vi "Dashboard Main.vi"() -> ()   [LabVIEW 2019]
uses:
  <vilib>/Utility/miscctls.llb/LVRowAndColumnTypeDef.ctl
  <vilib>/event_ctls.llb/eventvkey.ctl
  <vilib>/Rock Robotics/Network Tables/NT Read Numeric Array.vi
  <vilib>/Rock Robotics/WPI/Dashboard/WPI_DashboardLogging Global.vi
  <vilib>/Rock Robotics/Network Tables/NT Read Boolean.vi
panel:
  in  "Camera Settings Right":T1={"Frame Rate"=30, "Compression"=30, "Size"=1, "DB Camera Config"=FALSE} {"Frame Rate" scale=1.0..30.0; "Compression" scale=100.0..-1.0; "Size" items=["640x480", "320x240", "160x120"]}
  in  "Camera Name Right":string(combo)="No Camera Selection"
  out "Camera Perf":string
  in  "Camera Settings":T1={"Frame Rate"=30, "Compression"=30, "Size"=1, "DB Camera Config"=FALSE} {"Frame Rate" scale=1.0..30.0; "Compression" scale=100.0..-1.0; "Size" items=["640x480", "320x240", "160x120"]}
  in  "TCP":refnum<k5>
  in  "Rec Mode":enum32{"Stop", "Record", "Playback"}(radio)
  out "Robot IP":string
  out "Image Message":string="Timeout in Camera Communications"
  in  "Dashboard Tab":T2(tab)
  in  "FT to IN":bool
  out "Target Acquired":bool
  out "Vision Enabled":bool
  out "NT Connection":bool
  out "MotorChart R":cluster{"Numeric":dbl, "Numeric":dbl}(graph)
  out "MotorChart L":cluster{"Numeric":dbl, "Numeric":dbl}(graph)
  out "MotorSliders R":cluster{"MotorSlide1":dbl, "MotorSlide2":dbl} {"MotorSlide2" scale=-1.0..1.0 scale format="%#_2e"; "MotorSlide1" scale=-1.0..1.0 scale format="%#_2e"}
  out "MotorSliders L":cluster{"MotorSlide1":dbl, "MotorSlide2":dbl} {"MotorSlide2" scale=-1.0..1.0 scale format="%#_2e"; "MotorSlide1" scale=-1.0..1.0 scale format="%#_2e"}
  out "JS1 Z":dbl(slide) scale=-1.0..1.0 scale format="%#_2e"
  out "JS1 Graph":cluster{"X":dbl, "Y":dbl}[](graph)
  out "JS1 Buttons":T3
  out "JS2 Z":dbl(slide) scale=-1.0..1.0 scale format="%#_2e"
  out "JS2 Graph":cluster{"X":dbl, "Y":dbl}[](graph)
  out "JS2 Buttons":T3
  out "Mode":T4(ring)=enum."Auto Disabled"
  out "Right Camera Perf":cluster{"Bandwidth (Mbps)":dbl, "FPS":dbl}
  in  "Select Auto":string(combo)="Select Autonomous ..."
  out "Target Distance":dbl
  out "Camera Image Right":T5(plugin-control)
  out "Skew":dbl caption="DB/String 1"
  out "Area":dbl caption="DB/String 1"
  out "Offset X":dbl
  out "Offset Y":dbl
  out "Top RPM":dbl caption="DB/String 1"
  out "Bottom RPM":dbl caption="DB/String 1"
  in  "Test Slider":dbl(slide) scale=0.0..100.0 scale format="%#_3g"
  in  "On/Off":bool caption="Solenoid"
  in  "Test Name":u16(ring) items=["Select the test to run..."]
  in  "Test Tree":string(tree)
  in  "Motor":cluster{"Value":dbl, "Enable":bool} {"Value" scale=-1.0..1.0 scale format="%#_3g"}
  out "Progress":T6 {"Test Progress" scale=0.0..100.0}
  in  "Rev/Fwd":cluster{"Forward":bool, "Reverse":bool}
  in  "Test Ring":u16(ring) items=["Monochrome", "Color"]
  out "Cmd Status":string
  in  "Execute Command":bool
  in  "Command Params":string[][](table)
  in  "Command Selection":i32(listbox)
  in  "CheckList":i32(listbox)
  out "Tree":string(tree)
  out "Camera Image":T5(plugin-control)
  out "Background":bool
  in  "Camera Name":string(combo)="No Camera Selection"
  # "HW"
  # "HW"
  # "Drive Motors"
  # "Front"
  # "Operator 1"
  # "Operator 2"
  # "Right"
  # "Left"
  # "Back"
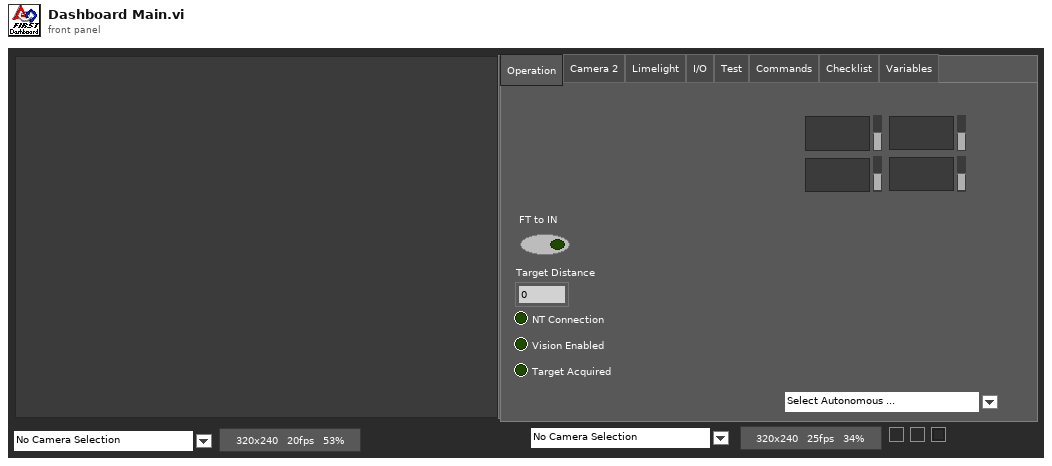
[diagram p1: front panel]
types:
  T1 = cluster{"Frame Rate":i32, "Compression":i32, "Size":u16, "DB Camera Config":bool}
  T2 = enum32{"Operation", "Camera 2", "Limelight", "I/O", "Test", "Commands", "Checklist", "Variables"}
  T3 = cluster{bool, bool, bool, bool, bool, bool, bool, bool, bool, bool, bool, bool}
  T4 = enum8{"Tele-Op Disabled", "Tele-Op Enabled", "Auto Disabled", "Auto Enabled", "Test Disabled", "Test Enabled", "Disconnected", "No Code", "E-Stop"}
  T5 = typedef "IMAQ Image.ctl" = refnum<image>
  T6 = cluster{"Test Progress":u8, "Test Progress Text":string}
  T7 = cluster{"Save Path":path, "Interval (s)":dbl, "Keep":i32}
  T8 = enum32{"Drive", "Camera", "Basic", "Custom", "Test", "Commands", "Checklist", "Variables"}
  T9 = typedef "Image Type" = u32
  T10 = cluster{"IDs":cluster{"RPC field ID":u16, "Unique ID":u16}, "String":string}
  T11 = cluster{"Camera Image":refnum<vi>, "Dashboard Tab":refnum<vi>, "Background":refnum<vi>, "Rec Mode":refnum<vi>, "Test Slider":refnum<vi>, "On/Off ":refnum<vi>, "Test Ring":refnum<vi>, "Rev/Fwd":refnum<vi>, "Test Name":refnum<vi>, "Motor":refnum<vi>, "Progress":refnum<vi>, "CheckList":refnum<vi>, "Tree":refnum<vi>, "Test Tree":refnum<vi>, "Command Params":refnum<vi>, "Command Selection":refnum<vi>, "Execute Command":refnum<vi>, "Cmd Status":refnum<vi>, "Camera Settings":refnum<vi>, "Camera Name":refnum<vi>, "Camera Perf":refnum<vi>, "Camera Settings Right":refnum<vi>, "Camera Name Right":refnum<vi>, "Camera Image Right":refnum<vi>}
  T12 = cluster{"Global Rectangle":i32[], "Contours":cluster{"Contour Type":u32, "ROI Type":u32, "Points":i32[]}[]}
  T13 = cluster{"Camera Name Right":string, string, "Saved DB Images Info":cluster{"Save Path":path, "Interval (s)":dbl, "Keep":i32}}
  T14 = cluster{"Error Strings":string, "Disable Counts":cluster{u16, u16}, "Rail Faults":cluster{u16, u16, u16}, "Robot IP":string, "DB Mode":u8, "Event Info":cluster{"Name":string, "Type":u8, "Number":u16, "Replay":u8}}
  T15 = cluster{"Storage":cluster{"Disk Free":u64, "RAM Block":u32, "RAM free":u32}, "CPU Utilization":cluster{"CPU % ISR":sgl, "CPU % Time Crit":sgl, "CPU % Timed Str":sgl, "CPU % High":sgl, "CPU % Above":sgl, "CPU % Normal":sgl, "CPU % Low":sgl}, "CAN":cluster{"% Bus Utilization":sgl, "Bus Off Cnt":u32, "TX_FIFO Full Cnt":u32, "Receive Error Cnt":u8, "Transmit Error Cnt":u8}, "HID":cluster{"HID Outputs":u32, "Rumble Low":u16, "Rumble High":u16}[]}
  T16 = cluster{"Status bits":cluster{"Test Mode":bool, "Autonomous":bool, "Enabled":bool, "Code Start":bool, "Brownout":bool, "Reserved 2":bool, "Reserved 3":bool, "E-Stop":bool}, "Code Trace":cluster{"Disabled":bool, "TeleOp":bool, "Auto":bool, "Test":bool}, "Controller Type":enum16{"unknown", "cRIO", "roboRio"}, "Code?":enum16{"unknown", "noCode", "code"}, "Battery V":dbl}
  T17 = cluster{"Control Bits":cluster{"TestMode":bool, "Autonomous":bool, "Enabled":bool, "FMS Present":bool, bool, bool, bool, "E-Stop":bool}, "Team Station ":u8, "Countdown":sgl, "Joystick Values":cluster{"Axes":dbl[], "Buttons":bool[], "POVs":i16[]}[]}
  T18 = cluster{"Axes":dbl[], "Buttons":bool[], "POVs":i16[]}[]
  T19 = cluster{"Axes":dbl[], "Buttons":bool[], "POVs":i16[]}
  T20 = cluster{"Buttons[0]":bool, "Buttons[1]":bool, "Buttons[2]":bool, "Buttons[3]":bool, "Buttons[4]":bool, "Buttons[5]":bool, "Buttons[6]":bool, "Buttons[7]":bool, "Buttons[8]":bool, "Buttons[9]":bool, "Buttons[10]":bool, "Buttons[11]":bool}
  T21 = cluster{"Camera Name":string, string, "Saved DB Images Info":cluster{"Save Path":path, "Interval (s)":dbl, "Keep":i32}}
  T22 = cluster{"Operation":enum16{"Update", "Clear"}, "Color Box":u32}[]
  T23 = typedef "eventvkey.ctl" = enum16{"ASCII", "Enter", "Return", "Shift", "Ctrl", "Alt", "Cmd", "Opt", "Caps", "NumLock", "Clear", "Break", "Up", "Down", "Left", "Right", "Insert", "Delete", "Home", "End", "PageUp", "PageDown", "Escape", "Help", "Pause", "ScrollLock", "F1", "F2", "F3", "F4", "F5", "F6", "F7", "F8", "F9", "F10", "F11", "F12", "F13", "F14", "F15", "F16", "F17", "F18", "F19", "F20", "F21", "F22", "F23", "F24", "Play", "VolumeUp", "VolumeDown", "Mute", "Two Byte Char"}
  T24 = cluster{"Image Size":bool, "Image Type":bool, "Pixel Value":bool, "ROI Information":bool, "Zoom Factor":bool}
  T25 = cluster{"Operation":enum16{"Update", "Clear"}, "Color Box":u32}
  T26 = typedef "LVRowAndColumnTypeDef.ctl" = cluster{"Row":i32, "Column":i32}
  T27 = cluster{"Shift":bool, "Ctrl":bool, "Alt":bool, "Cmd":bool, "Opt":bool}
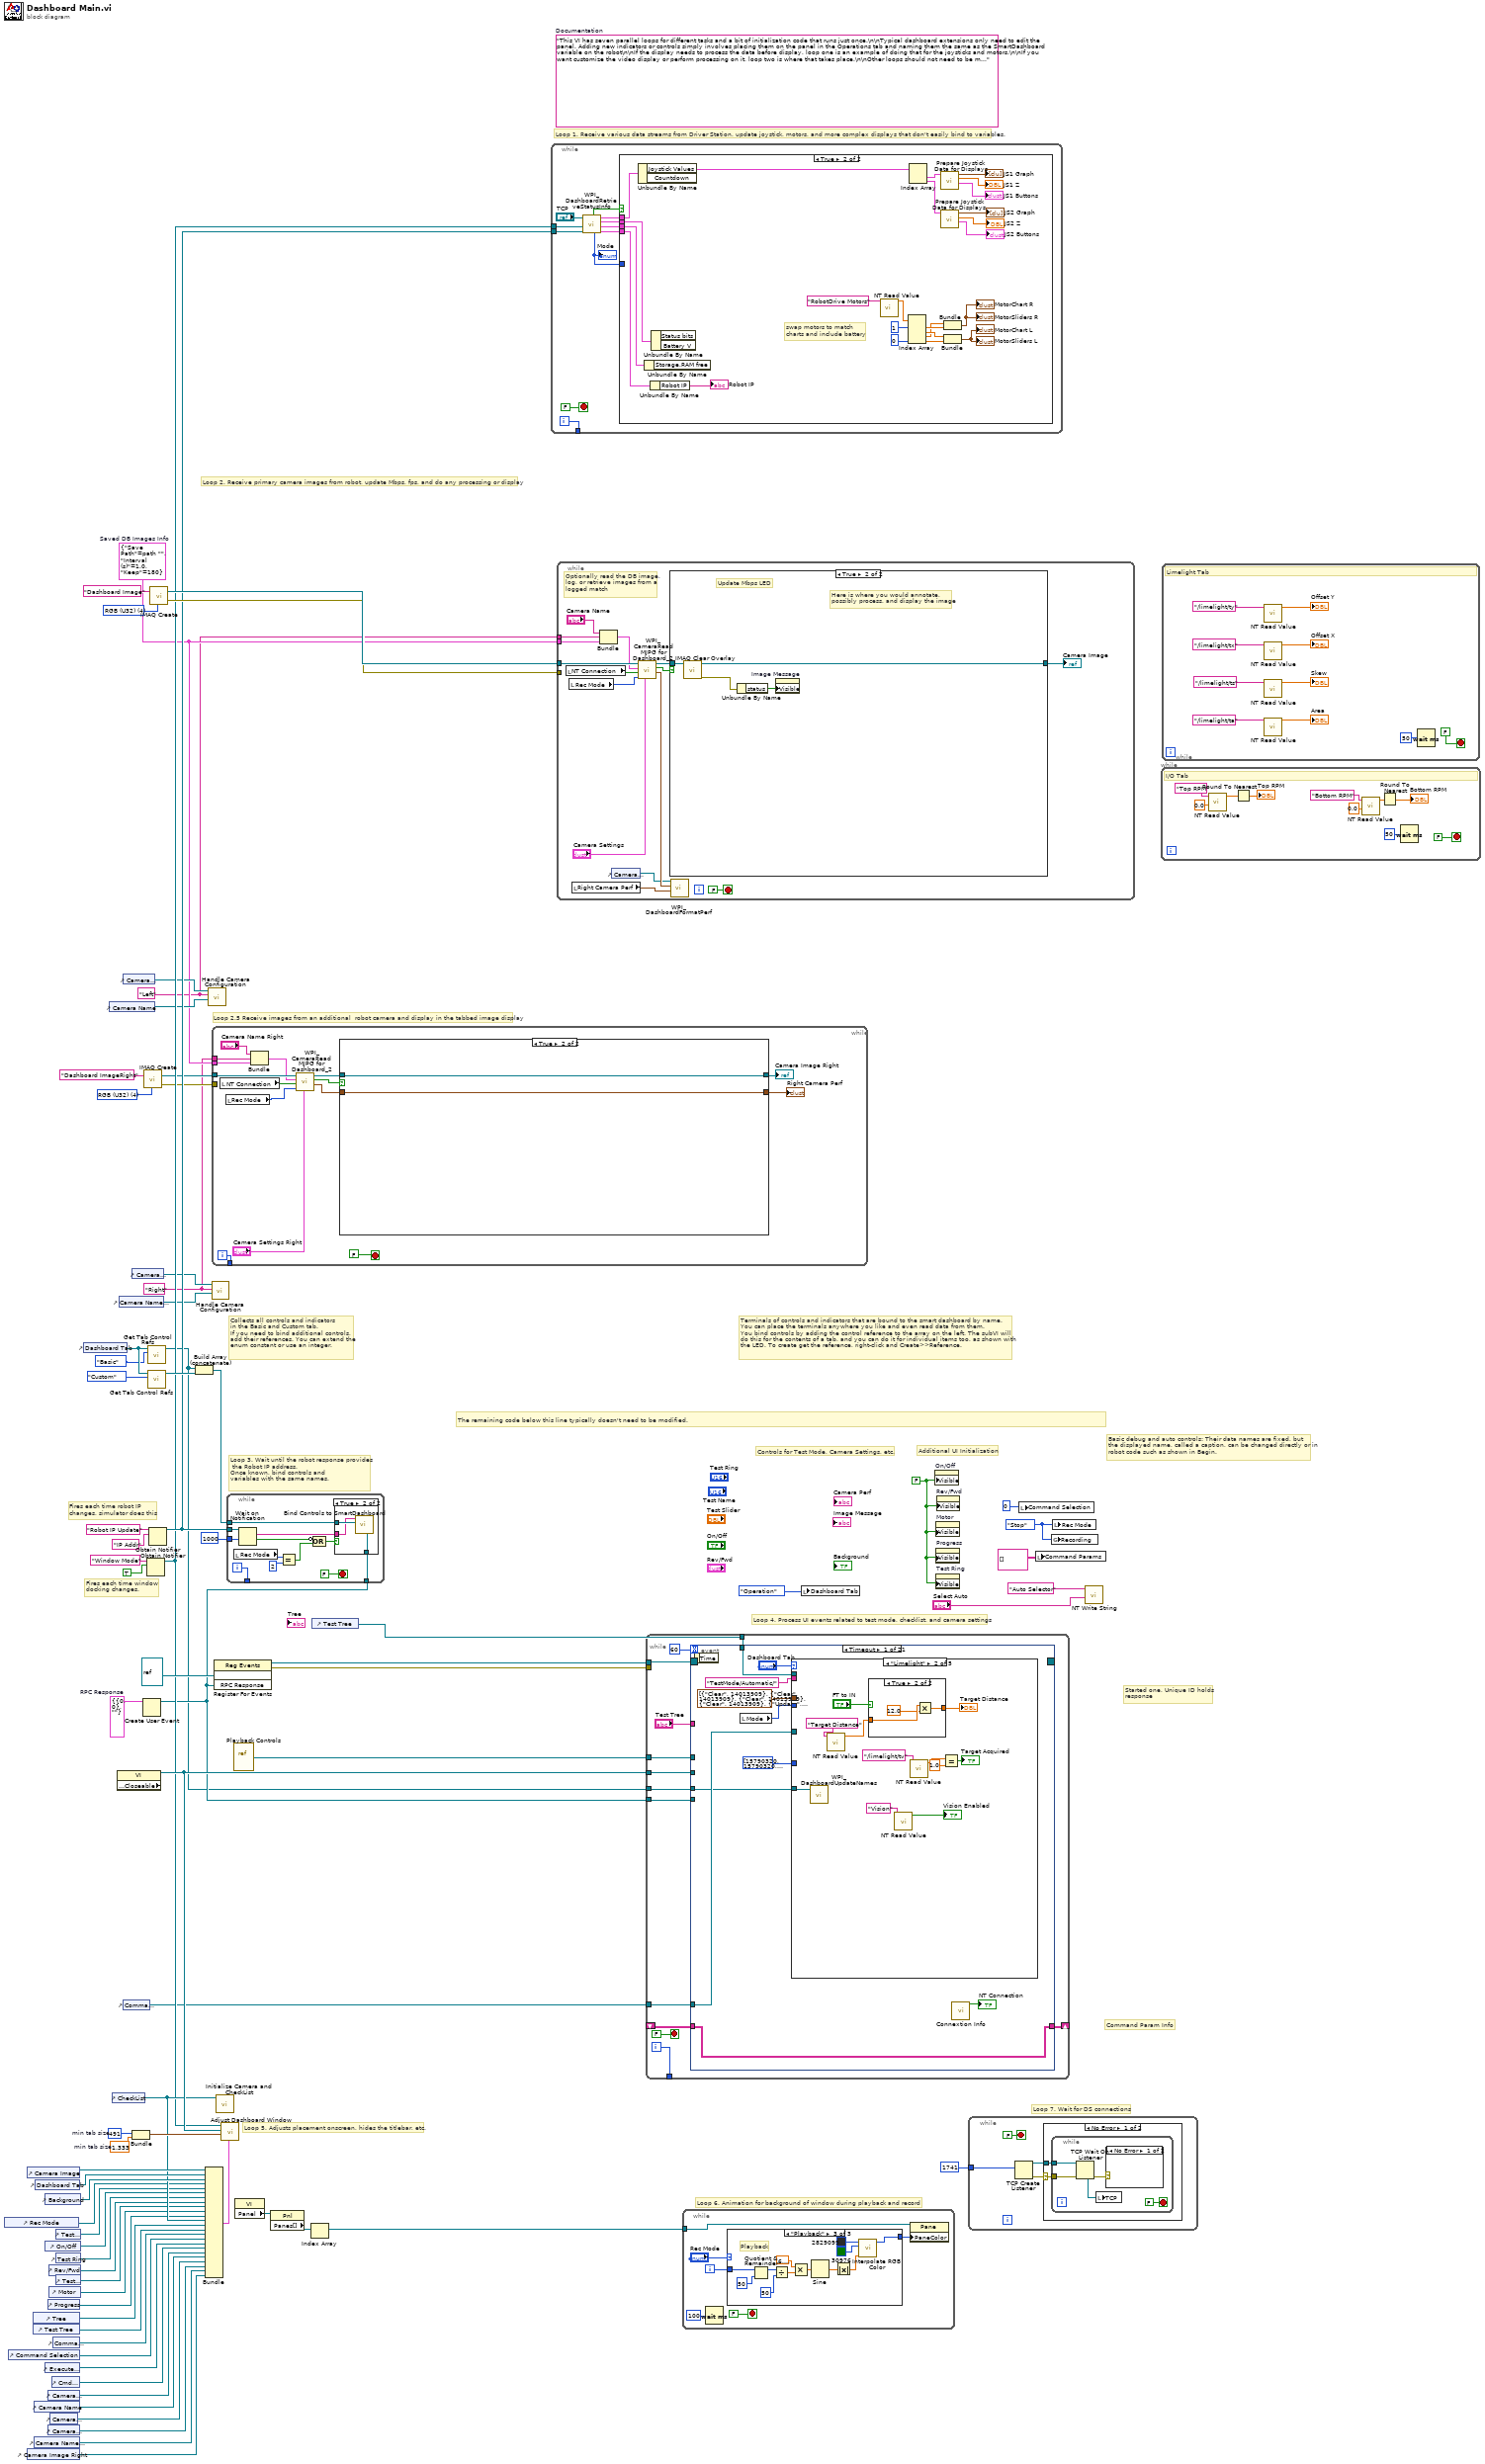
[diagram p0: block diagram]
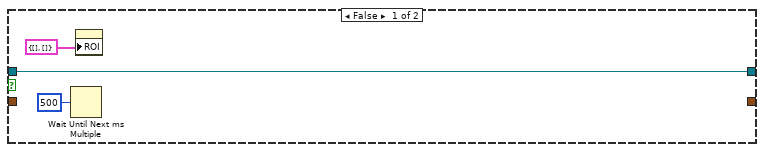
[diagram p2: hidden frame]
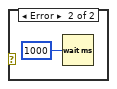
[diagram p3: hidden frame]
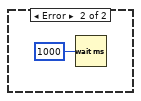
[diagram p4: hidden frame]
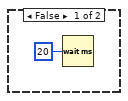
[diagram p5: hidden frame]
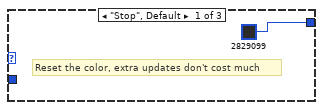
[diagram p6: hidden frame]
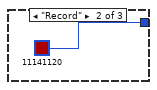
[diagram p7: hidden frame]
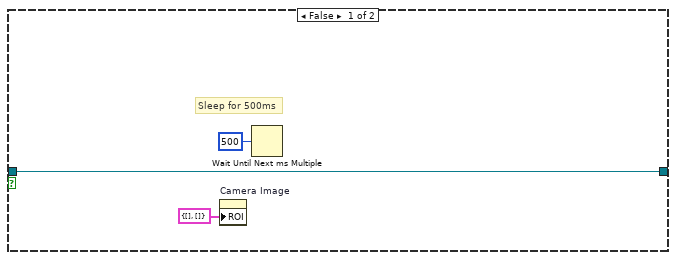
[diagram p9: hidden frame]
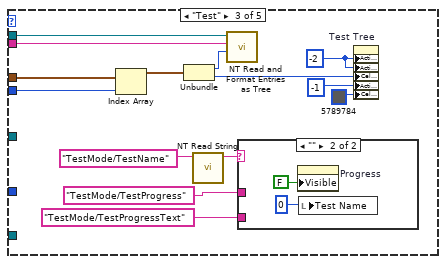
[diagram p12: hidden frame]
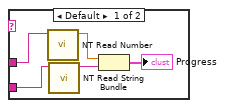
[diagram p13: hidden frame]
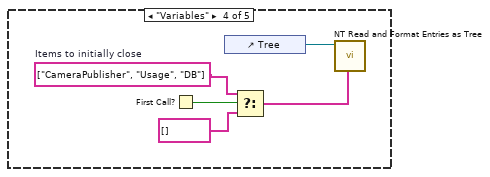
[diagram p14: hidden frame]
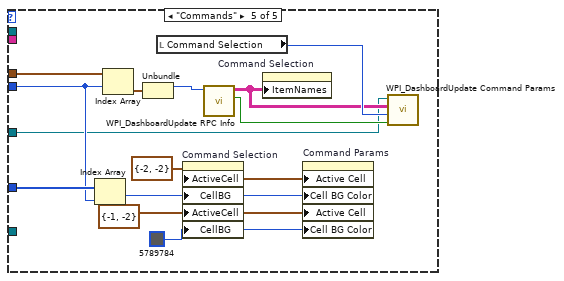
[diagram p15: hidden frame]
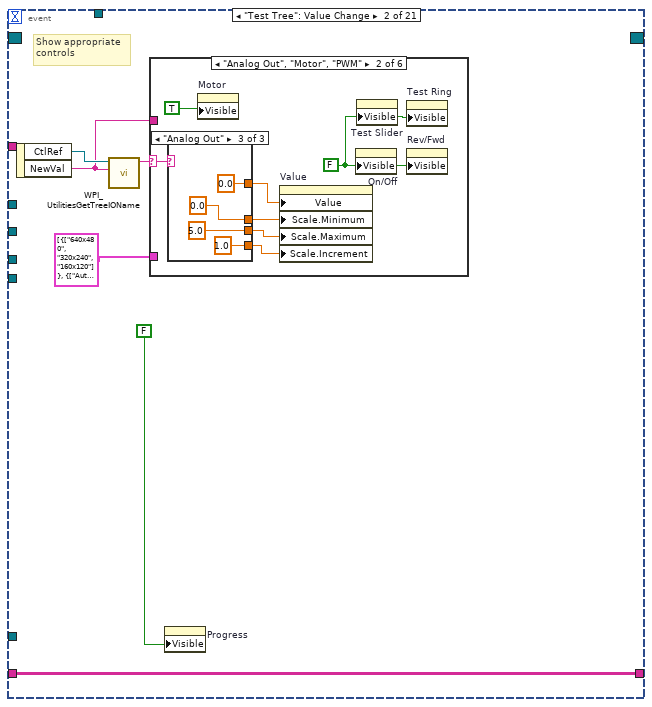
[diagram p16: hidden frame]
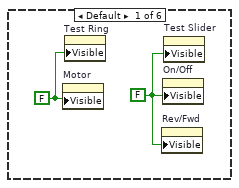
[diagram p17: hidden frame]
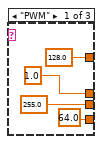
[diagram p18: hidden frame]
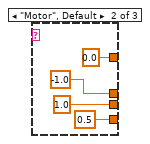
[diagram p19: hidden frame]
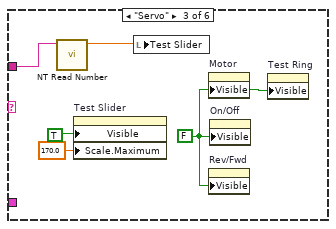
[diagram p20: hidden frame]
diagram:
  w4 = T7 {"Save Path"=path "", "Interval (s)"=1.0, "Keep"=180}  # Saved DB Images Info
  w3 = "Right"
  w2 = "Left"
  w14 = T9 4 items=["Grayscale (U8)", "Grayscale (I16)", "Grayscale (SGL)", "Complex (CSG)", "RGB (U32)", "HSL (U32)", "RGB (U64)"] ("Image Type")
  w30 = T10 {"IDs"={"RPC field ID"=0, "Unique ID"=0}, "String"=""}  # RPC Response
  w52 = 491  # min tab size
  w51 = 1.333  # min tab size
  w59 = enum32{"Stop", "Record", "Playback"}."Stop" ("Rec Mode")
  w36 = FALSE ("Visible")
  (unwired) "This VI has seven parallel loops for different tasks and a bit of initialization code that runs just once.\n\nTypical dashboard extensions only need to edit the panel. Adding new indicators or controls simply involves placing them on the panel in the Operations tab and naming them the same as the SmartDashboard variable on the robot\n\nIf the display needs to process the data before display, loop one is an example of doing that for the joysticks and motors.\n\nIf you want customize the video display or perform processing on it, loop two is where that takes place.\n\nOther loops should not need to be modified. They are pretty standard, and document the task they perform."  # Documentation
  w76 = T9 4 items=["Grayscale (U8)", "Grayscale (I16)", "Grayscale (SGL)", "Complex (CSG)", "RGB (U32)", "HSL (U32)", "RGB (U64)"] ("Image Type")
  # "Loop 2.5 Receive images from an additional  robot camera and display in the tabbed image display"
  # "Command Param Info"
  # "Started one, Unique ID holds\nresponse"
  # "Loop 7. Wait for DS connections"
  # "Basic debug and auto controls: Their data names are fixed, but\nthe displayed name, called a caption, can be changed directly or in\nrobot code such as shown in Begin."
  # "Controls for Test Mode, Camera Settings, etc."
  # "Additional UI Initialization"
  # "Loop 6. Animation for background of window during playback and record"
  # "Fires each time robot IP\nchanges, simulator does this"
  # "Fires each time window\ndocking changes."
  # "Collects all controls and indicators\nin the Basic and Custom tab.\nIf you need to bind additional controls,\nadd their references. You can extend the\nenum constant or use an integer."
  # "The remaining code below this line typically doesn't need to be modified."
  # "Loop 4. Process UI events related to test mode, checklist, and camera settings"
  # "Terminals of controls and indicators that are bound to the smart dashboard by name.\nYou can place the terminals anywhere you like and even read data from them.\nYou bind controls by adding the control reference to the array on the left. The subVI will\ndo this for the contents of a tab, and you can do it for individual items too, as shown with\nthe LED. To create get the reference, right-click and Create>>Reference."
  # "Loop 3. Wait until the robot response provides\n the Robot IP address.\nOnce known, bind controls and\nvariables with the same names."
  # "Loop 5. Adjusts placement onscreen, hides the titlebar, etc."
  # "Loop 1. Receive various data streams from Driver Station, update joystick, motors, and more complex displays that don't easily bind to variables."
  # "Loop 2. Receive primary camera images from robot, update Mbps, fps, and do any processing or display"
  n1 = control-ref of="Rec Mode"() -> (w42:refnum<vi>)
  n2 = control-ref of="Command Selection"() -> (w29:refnum<vi>)
  n3 = control-ref of="Camera Image Right"() -> (w7:refnum<vi>)
  n4 = control-ref of="Camera Image"() -> (w54:refnum<vi>)
  n5 = control-ref of="Tree"() -> (w46:refnum<vi>)
  n6 = control-ref of="Test Tree"() -> (w45:refnum<vi>)
  n7 = control-ref of="Camera Name"() -> (w20:refnum<vi>)
  n8 = control-ref of="Camera Name Right"() -> (w8:refnum<vi>)
  n9 = control-ref of="Dashboard Tab"() -> (w53:refnum<vi>)
  n10 = control-ref of="Execute Command"() -> (w31:refnum<vi>)
  n11 = control-ref of="Background"() -> (w49:refnum<vi>)
  n12 = control-ref of="On/Off"() -> (w40:refnum<vi>)
  n13 = control-ref of="Progress"() -> (w37:refnum<vi>)
  n14 = control-ref of="Camera Settings"() -> (w21:refnum<vi>)
  n15 = control-ref of="Camera Settings Right"() -> (w9:refnum<vi>)
  n16 = control-ref of="Rev/Fwd"() -> (w38:refnum<vi>)
  n17 = control-ref of="Motor"() -> (w43:refnum<vi>)
  n18 = control-ref of="Camera Perf"() -> (w19:refnum<vi>)
  n19 = control-ref of="Cmd Status"() -> (w25:refnum<vi>)
  n20 = control-ref of="Command Params"() -> (w32:refnum<vi>)
  n21 = control-ref of="Test Slider"() -> (w41:refnum<vi>)
  n22 = control-ref of="Test Ring"() -> (w39:refnum<vi>)
  n23 = control-ref of="Test Name"() -> (w44:refnum<vi>)
  n24 = control-ref of="Dashboard Tab"() -> (w57:refnum<vi>)
  n25 = control-ref of="Camera Name"() -> (w22:refnum<vi>)
  n26 = control-ref of="CheckList"() -> (w47:refnum<vi>)
  n27 = property class="VI" props=["Front Panel.Closeable"]() -> (reference out=w58:refnum<vi>)  [unwired: 2 in, 2 out]
  n28 = control-ref of="Camera Name Right"() -> (w10:refnum<vi>)
  n29 = control-ref of="Camera Settings"() -> (w23:refnum<vi>)
  n30 = control-ref of="Command Params"() -> (w24:refnum<vi>)
  n31 = control-ref of="Camera Settings Right"() -> (w11:refnum<vi>)
  n32 = Bundle("min tab size"=w52, "min tab size"=w51) -> (w50:cluster{"min tab size":i32, "min tab size":dbl})  [unwired: 1 in]
  n33 = Create User Event(user event datatype=w30) -> (user event=w26:refnum<user-event>)  [unwired: 1 in, 1 out]
  n34 = call "IMAQ Create"("Image Name"="Dashboard ImageRight", "Image Type"=w14) -> ("New Image"=w13:T5, "error out"=w12:errorcluster)  [unwired: 2 in, 1 out]
  n35 = Obtain Notifier(name (unnamed)="Window Mode", notification data type=TRUE) -> (notifier out=w34:refnum<notifier>)  [unwired: 2 in, 2 out]
  n36 = call <vilib>:"Get Tab Control Refs.vi"("Page Index"=T8."Basic" ("Dashboard Tab"), "TabControl in"=w57) -> ("ControlsOnPage"=w18:refnum<vi>[])  [unwired: 9 in]
  n37 = call <vilib>:"Get Tab Control Refs.vi"("Page Index"=T8."Custom" ("Dashboard Tab"), "TabControl in"=w57) -> ("ControlsOnPage"=w56:refnum<vi>[])  [unwired: 9 in]
  n38 = Obtain Notifier(name (unnamed)="Robot IP Update", notification data type="IP Addr" ("name (unnamed)")) -> (notifier out=w35:refnum<notifier>)  [unwired: 2 in, 2 out]
  n39 = call "IMAQ Create"("Image Name"="Dashboard Image", "Image Type"=w76) -> ("New Image"=w74:T5, "error out"=w73:errorcluster)  [unwired: 2 in, 1 out]
  n40 = Build Array (concatenate)(w18, w56) -> (w55:refnum<vi>[])
  n41 = Bundle("Camera Image"=w54, "Dashboard Tab"=w53, "Background"=w49, "Rec Mode"=w42, "Test Slider"=w41, "On/Off"=w40, "Test Ring"=w39, "Rev/Fwd"=w38, "Test Name"=w44, "Motor"=w43, "Progress"=w37, "CheckList"=w47, "Tree"=w46, "Test Tree"=w45, "Command Params"=w32, "Command Selection"=w29, "Execute Command"=w31, "Cmd Status"=w25, "Camera Settings"=w21, "Camera Name"=w20, "Camera Perf"=w19, "Camera Settings Right"=w9, "Camera Name Right"=w8, "Camera Image Right"=w7) -> (w48:T11)  [unwired: 1 in]
  n42 = call "Handle Camera Configuration.vi"("CameraNameRef"=w22, "Display Name"=w2, "ClusterRef"=w23) -> ()  [unwired: 9 in]
  n43 = call "Handle Camera Configuration.vi"("CameraNameRef"=w10, "Display Name"=w3, "ClusterRef"=w11) -> ()  [unwired: 9 in]
  n44 = while {
    tunnel: w13 -> [w91]
    tunnel: w12 -> [_]
    tunnel: [w86] -> _
    tunnel: w4 -> [w83]
    tunnel: w3 -> [w80]
    i -> [w86]
    stop <- FALSE stop-if-true
    n45 = local read "NT Connection"() -> (w84:bool)
    n46 = local read "Rec Mode"() -> (w90:enum32{"Stop", "Record", "Playback"})
    n47 = Bundle("Camera Name Right"="Camera Name Right", w80, "Saved DB Images Info"=w83) -> (w82:T13)  [unwired: 1 in]
    n48 = call <vilib>:"WPI_CameraRead MJPG for Dashboard_2.vi"("Camera Settings"="Camera Settings Right", "Rec Mode"=w90, "NT Connection"=w84, "Capture Info"=w82, "Image in"=w91) -> ("perf info"=w78:cluster{"Bandwidth (Mbps)":dbl, "fps":dbl}, "Active"=w85:bool, "Image\\ out"=w88:T5)  [unwired: 4 in]
    n49 = case shown="True" w85 {
      tunnel: w88 -> [w93 w95]
      tunnel: [w93 w95] -> w77
      tunnel: [_ w96] -> w79
      tunnel: w78 -> [_ w96]
      frame False {
        n50 = Wait Until Next ms Multiple(millisecond multiple=u32 500) -> ()  [unwired: 1 out]
        n51 = property on="Camera Image Right" class="ImageControl"("ROI"=T12 {"Global Rectangle"=[], "Contours"=[]}) -> ()  [unwired: 2 in, 2 out]
      }
      frame True {
      }
    }
    "Right Camera Perf" <- w79
    "Camera Image Right" <- w77
  }
  n52 = register-events(refnum<vi> refnum, w26) -> (reference out=w63:refnum<event-registration>, error out=w62:errorcluster)  [unwired: 2 in]
  n53 = call "Initialize Camera and CheckList.vi"("ListBox in"=w47) -> ()  [unwired: 11 in]
  n54 = call "Adjust Dashboard Window.vi"("Sizing Refnums"=w48, "Size Constraints"=w50, "VI"=w58, "WIn Mode"=w34) -> ()  [unwired: 8 in]
  n55 = while {
    tunnel: w55 -> [w108]
    tunnel: w35 -> [w106]
    tunnel: [w104] -> _
    tunnel: u32 1000 ("milliseconds to wait") -> [w103]
    tunnel: w26 -> [w97]
    i -> [w104]
    stop <- FALSE stop-if-true
    n56 = local read "Rec Mode"() -> (w99:enum32{"Stop", "Record", "Playback"})
    n57 = Wait on Notification(notifier=w106, timeout in ms (-1)=w103) -> (notification=w105:string, timed out?=w101:bool)  [unwired: 2 in, 2 out]
    n58 = Equal?(x=w99, y=u16 2 ("Rec Mode")) -> (x = y?=w100:bool)
    n59 = Compound Arithmetic op=OR(invert w101, w100) -> (w102:bool)
    n60 = case shown="True" w102 {
      tunnel: w108 -> [_ w111]
      tunnel: w105 -> [_ w110]
      tunnel: w97 -> [_ w109]
      frame False {
      }
      frame True {
        n61 = call <vilib>:"Bind Controls to SmartDashboard.vi"("RPC ref"=w109, "Bound Control Refs"=w111, "Server IP Address"=w110) -> ()  [unwired: 9 in]
      }
    }
  }
  n62 = vi-ref "Playback Controls.vi"() -> (w64:refnum<vi>)
  n63 = property class="VI"() -> ("Panel"=w66:refnum<vi>)  [unwired: 2 in, 2 out]
  n64 = property class="Pnl"(reference=w66) -> ("Panes[]"=w67:refnum<vi>[])  [unwired: 1 in, 2 out]
  n65 = Index Array(array=w67) -> (element=w65:refnum<vi>)  [unwired: 1 in]
  n66 = control-ref of="Test Tree"() -> (w68:refnum<vi>)
  n67 = while {
    tunnel: [w121] -> _
    tunnel: w35 -> [w115]
    tunnel: w34 -> [w112]
    i -> [w121]
    stop <- FALSE stop-if-true
    n68 = call <vilib>:"WPI_DashboardRetrieveStatusInfo.vi"("Binding Refnum"=w115, "Window Mode Notifier"=w112, "TCP Cnx"="TCP") -> ("Power and Errors"=w116:T14, "Robot Metrics"=w119:T15, "Status Info"=w120:T16, "Control Info"=w117:T17, "Robot Mode"=w114:T4, "Process?"=w118:bool)  [unwired: 3 in]
    "Mode" <- w114
    n69 = case shown="True" w118 {
      tunnel: w120 -> [_ w147]
      tunnel: w119 -> [_ w146]
      tunnel: w117 -> [_ w145]
      tunnel: w116 -> [_ w144]
      tunnel: w114 -> [_ _]
      frame False {
        n70 = Wait (ms)(milliseconds to wait=u32 20) -> ()  [unwired: 1 out]
      }
      frame True {
        # "swap motors to match\ncharts and include battery"
        n71 = Unbundle By Name(w145) -> ("Joystick Values"=w135:T18)  [unwired: 1 out]
        n72 = Unbundle By Name(w146) -> ()  [unwired: 1 out]
        n73 = Unbundle By Name(w144) -> ("Robot IP"=→"Robot IP":string)
        n74 = Unbundle By Name(w147) -> ()  [unwired: 2 out]
        n75 = call-poly <vilib>:"NT Read Value.vi"("Name"="RobotDrive Motors") -> ("Numeric Array"=w125:dbl[])  [unwired: 9 in, 1 out]
        n76 = Index Array(array=w125, index #1=1, index #4=0) -> (element #1=w139:dbl, element #2=w140:dbl, element #3=w138:dbl, element #4=w143:dbl)  [unwired: 2 in]
        n77 = Index Array(array=w135) -> (element #1=w134:T19, element #2=w130:T19)  [unwired: 2 in]
        n78 = call "Prepare Joystick Data for Displays.vi"("Joystick Values"=w130) -> ("Buttons"=→"JS2 Buttons":T20, "Z Axis"=→"JS2 Z":dbl, "Cartesian Data"=→"JS2 Graph":cluster{"X axis":dbl, "X axis":dbl}[])  [unwired: 8 in]
        n79 = call "Prepare Joystick Data for Displays.vi"("Joystick Values"=w134) -> ("Buttons"=→"JS1 Buttons":T20, "Z Axis"=→"JS1 Z":dbl, "Cartesian Data"=→"JS1 Graph":cluster{"X axis":dbl, "X axis":dbl}[])  [unwired: 8 in]
        n80 = Bundle("Numeric"=w138, "Numeric"=w139) -> (→"MotorChart R" →"MotorSliders R":cluster{"Numeric":dbl, "Numeric":dbl})  [unwired: 1 in]
        n81 = Bundle("Numeric"=w140, "Numeric"=w143) -> (→"MotorChart L" →"MotorSliders L":cluster{"Numeric":dbl, "Numeric":dbl})  [unwired: 1 in]
      }
    }
  }
  n82 = while {
    tunnel: w74 -> [w161]
    tunnel: w73 -> [_]
    tunnel: w4 -> [w155]
    tunnel: w2 -> [w152]
    stop <- FALSE stop-if-true
    # "Optionally read the DB image,\nlog, or retrieve images from a\nlogged match"
    n83 = local read "NT Connection"() -> (w156:bool)
    n84 = local read "Rec Mode"() -> (w158:enum32{"Stop", "Record", "Playback"})
    n85 = local read "Right Camera Perf"() -> (w150:cluster{"Bandwidth (Mbps)":dbl, "FPS":dbl})
    n86 = Bundle("Camera Name"="Camera Name", w152, "Saved DB Images Info"=w155) -> (w154:T21)  [unwired: 1 in]
    n87 = control-ref of="Camera Perf"() -> (w149:refnum<vi>)
    n88 = call <vilib>:"WPI_CameraRead MJPG for Dashboard_2.vi"("Camera Settings"="Camera Settings", "Rec Mode"=w158, "NT Connection"=w156, "Capture Info"=w154, "Image in"=w161) -> ("perf info"=w151:cluster{"Bandwidth (Mbps)":dbl, "fps":dbl}, "Active"=w159:bool, "Image\\ out"=w160:T5)  [unwired: 4 in]
    n89 = case shown="True" w159 {
      tunnel: w160 -> [w164 w167]
      tunnel: [w164 w166] -> w148
      frame False {
        # "Sleep for 500ms"
        n90 = property on="Camera Image" class="ImageControl"("ROI"=T12 {"Global Rectangle"=[], "Contours"=[]}) -> ()  [unwired: 2 in, 2 out]
        n91 = Wait Until Next ms Multiple(millisecond multiple=u32 500) -> ()  [unwired: 1 out]
      }
      frame True {
        # "Here is where you would annotate,\npossibly process, and display the image"
        # "Update Mbps LED"
        n92 = call "IMAQ Clear Overlay"("Image"=w167) -> ("error out"=w168:errorcluster, "Image Out"=w166:T5)  [unwired: 2 in, 7 out]
        n93 = Unbundle By Name(w168) -> ("status"=w169:bool)
        n94 = property on="Image Message" class="Str"("Visible"=w169) -> ()  [unwired: 2 in, 2 out]
      }
    }
    "Camera Image" <- w148
    n95 = call <vilib>:"WPI_DashboardFormatPerf.vi"("Right Camera Perf"=w150, "Performance"=w151, "String in"=w149) -> ()  [unwired: 9 in]
  }
  n96 = while {
    tunnel: [w179] -> _
    tunnel: w68 -> [w178]
    tunnel: w64 -> [w177]
    tunnel: w63 -> [w176]
    tunnel: w62 -> [_]
    tunnel: w58 -> [w175]
    tunnel: w26 -> [w174]
    tunnel: w24 -> [w173]
    shift-right: [w172] -> _
    shift-left: _ -> [w171]
    tunnel: w18 -> [w170]
    i -> [w179]
    stop <- FALSE stop-if-true
    n97 = event shown="[0] Timeout" {
      selector: w176 -> [_ _ _ _ _ _ _ _ _ _ _ _ _ _ _ _ _ _ _ _ _]
      dyn-events: [_ _ _ _ _ _ _ _ _ _ _ _ _ _ _ _ w453 _ _ _ _] -> _
      timeout: u32 60 ("milliseconds to wait") -> [_ _ _ _ _ _ _ _ _ _ _ _ _ _ _ _ _ _ _ _ _]
      tunnel: w178 -> [w191 _ _ _ _ _ _ _ _ _ _ _ _ _ _ _ _ _ _ _ _]
      tunnel: "Test Tree" -> [_ _ _ _ _ _ _ _ _ _ _ w420 w428 w430 w434 w442 _ _ _ _ _]
      tunnel: w177 -> [_ _ _ _ _ _ _ _ _ _ _ _ _ _ _ _ w455 _ w473 _ _]
      tunnel: w175 -> [_ _ _ _ _ _ _ _ _ _ _ _ _ _ _ _ w451 _ _ _ _]
      tunnel: w174 -> [_ _ _ _ _ _ _ _ _ _ _ _ _ _ _ _ w449 _ _ _ _]
      tunnel: w173 -> [w186 _ _ _ _ _ w371 _ _ _ _ _ _ _ _ _ _ _ _ _ _]
      tunnel: [w185 w248 w350 w355 w364 w368 w369 w378 w388 w395 w407 w419 w426 w429 w433 w441 w448 w468 w470 w474 w487] -> w172
      tunnel: w171 -> [w185 w248 w350 w355 w364 w368 w369 _ _ w395 w407 w419 w426 w429 w433 w441 w448 w468 w470 w474 w487]
      tunnel: w170 -> [w183 _ _ _ _ _ _ _ _ _ _ _ _ _ _ _ _ _ _ _ _]
      event Timeout {
        n98 = event-data() -> ()  [unwired: 1 in, 1 out]
        n99 = local read "Mode"() -> (w188:T4)
        n100 = case shown="\"Limelight\"" "Dashboard Tab" {
          tunnel: w191 -> [_ _ w221 _ _]
          tunnel: "TestMode/Automatic/" ("Name Pattern") -> [_ _ w220 _ _]
          tunnel: T22 [{"Operation"=enum."Clear", "Color Box"=14013909}, {"Operation"=enum."Clear", "Color Box"=14013909}, {"Operation"=enum."Clear", "Color Box"=14013909}, {"Operation"=enum."Clear", "Color Box"=14013909}, {"Operation"=enum."Update", "Color Box"=14013909}, {"Operation"=enum."Update", "Color Box"=16777215}, {"Operation"=enum."Clear", "Color Box"=14013909}, {"Operation"=enum."Clear", "Color Box"=14013909}, {"Operation"=enum."Clear", "Color Box"=14013909}] -> [_ _ w213 _ w241]
          tunnel: w188 -> [_ _ w212 _ w240]
          tunnel: u32[] [15790320, 15790320, 15790320, 15790320, 16777215, 16777215, 15790320, 15790320, 15790320] -> [_ _ _ _ w246]
          tunnel: w186 -> [_ _ _ _ w234]
          tunnel: w183 -> [_ w203 _ _ _]
          frame "I/O", Default {
          }
          frame "Limelight" {
            n101 = call <vilib>:"WPI_DashboardUpdateNames.vi"("Controls on Tab"=w203) -> ()  [unwired: 11 in]
            n102 = call-poly <vilib>:"NT Read Value.vi"("Name"="Target Distance") -> ("Numeric"=w201:dbl)  [unwired: 9 in, 1 out]
            n103 = case shown="True" "FT to IN" {
              tunnel: w201 -> [w204 w206]
              tunnel: [w204 w207] -> w202
              frame False {
              }
              frame True {
                n104 = Multiply(x=w206, y=12.0) -> (x*y=w207:dbl)
              }
            }
            "Target Distance" <- w202
            n105 = call-poly <vilib>:"NT Read Value.vi"("Name"="Vision") -> ("Boolean"=→"Vision Enabled":bool)  [unwired: 9 in, 1 out]
            n106 = call-poly <vilib>:"NT Read Value.vi"("Name"="/limelight/tv") -> ("Numeric"=w197:dbl)  [unwired: 9 in, 1 out]
            n107 = Equal?(x=w197, y=1.0) -> (x = y?=→"Target Acquired":bool)
          }
          frame "Test" {
            w219 = -2 ("Active Item:Row Number")
            n108 = Index Array(array=w213, index=w212) -> (element=w214:T25)
            n109 = Unbundle(w214) -> ("Operation"=w215:enum16{"Update", "Clear"}, "Color Box"=w216:u32)
            n110 = call <vilib>:"NT Read String.vi"("Name"="TestMode/TestName") -> ("String"=w210:string)  [unwired: 9 in, 1 out]
            n111 = call <vilib>:"NT Read and Format Entries as Tree.vi"("Operation"=w215, "Name Pattern"=w220, "Tree Refnum"=w221) -> ()  [unwired: 7 in, 2 out]
            n112 = case shown="\"\"" w210 {
              tunnel: "TestMode/TestProgress" ("Name") -> [w223 _]
              tunnel: "TestMode/TestProgressText" ("Name") -> [w222 _]
              frame Default {
                n113 = call <vilib>:"NT Read Number.vi"("Name"=w223) -> ("Numeric"=w224:dbl)  [unwired: 9 in, 1 out]
                n114 = call <vilib>:"NT Read String.vi"("Name"=w222) -> ("String"=w225:string)  [unwired: 9 in, 1 out]
                n115 = Bundle("Numeric"=w224, "String"=w225) -> (→"Progress":cluster{"Numeric":dbl, "String":string})  [unwired: 1 in]
              }
              frame "" {
                n116 = property on="Progress" class="Clust (strict)"("Visible"=FALSE) -> ()  [unwired: 2 in, 2 out]
                n117 = local write "Test Name"(u16 0) -> ()
              }
            }
            n118 = property on="Test Tree" class="Tree (strict)"("Active Item Row Number"=w219, "ActiveColNum"=w219, "CellBG"=w216, "Active Item Row Number"=-1 ("Active Item:Row Number"), "CellBG"=u32 5789784 ("Color Box")) -> ()  [unwired: 2 in, 2 out]
          }
          frame "Variables" {
            w231 = string[] ["CameraPublisher", "Usage", "DB"]  # Items to initially close
            n119 = First Call?() -> (First Call?: T/F=w232:bool)
            n120 = control-ref of="Tree"() -> (w233:refnum<vi>)
            n121 = Select(t=w231, s=w232, f=string[] []) -> (s? t:f=w229:string[])
            n122 = call <vilib>:"NT Read and Format Entries as Tree.vi"("Tags to  Close"=w229, "Tree Refnum"=w233) -> ()  [unwired: 8 in, 2 out]
          }
          frame "Commands" {
            w242 = u32 5789784 ("Color Box")
            w243 = T26 {"Row"=-1, "Column"=-2} ("Active Cell:Active Cell")
            w245 = T26 {"Row"=-2, "Column"=-2} ("Active Cell:Active Cell")
            n123 = Index Array(array=w246, index=w240) -> (element=w244:u32)
            n124 = Index Array(array=w241, index=w240) -> (element=w239:T25)
            n125 = Unbundle(w239) -> ("Operation"=w238:enum16{"Update", "Clear"})  [unwired: 1 out]
            n126 = local read "Command Selection"() -> (w237:i32)
            n127 = property on="Command Selection" class="MCListbox (strict)"("ActiveCell"=w245, "CellBG"=w244, "ActiveCell"=w243, "CellBG"=w242) -> ()  [unwired: 2 in, 2 out]
            n128 = call <vilib>:"WPI_DashboardUpdate RPC Info.vi"("Operation"=w238) -> ("update"=w236:bool, "commands"=w235:string[][])  [unwired: 9 in]
            n129 = property on="Command Selection" class="MCListbox (strict)"("ItemNames"=w235) -> ()  [unwired: 2 in, 2 out]
            n130 = property on="Command Params" class="Tbl (strict)"("Active Cell"=w245, "Cell BG Color"=w244, "Active Cell"=w243, "Cell BG Color"=w242) -> ()  [unwired: 2 in, 2 out]
            n131 = call <vilib>:"WPI_DashboardUpdate Command Params.vi"("Update"=w236, "NewVal"=w237, "Commands"=w235, "Param Tbl"=w234) -> ()  [unwired: 7 in, 1 out]
          }
        }
        n132 = call <vilib>:"Connextion Info.vi"() -> ("Connected"=→"NT Connection":bool)  [unwired: 10 in, 1 out]
      }
      event "Test Tree": Value Change {
        # "Show appropriate\ncontrols"
        n133 = event-data() -> ("CtlRef"=w251:refnum<vi>, "NewVal"=w249:string)  [unwired: 1 in]
        n134 = call <vilib>:"WPI_UtilitiesGetTreeIOName.vi"("NewVal"=w249, "TreeControl in"=w251) -> ("I/O Name"=w252:string)  [unwired: 9 in]
        n135 = case shown="\"Analog Out\", \"Motor\", \"PWM\"" w252 {
          selector: w252 -> [_ w259 _ w281 w290 _]
          tunnel: w249 -> [_ _ w278 w280 _ w297]
          tunnel: cluster{string[]}[] [{["640x480", "320x240", "160x120"]}, {["Auto", "Fixed indoor", "Fixed outdoor 1", "Fixed outdoor 2", "Fixed fluorescent 1", "Fixed fluorescent 2", "Hold current"]}, {["Auto", "Flicker-free 50 Hz", "Flicker-free 60 Hz", "Hold current"]}, {["None", "Prioritize frame rate", "Prioritize image quality"]}, {["Monochrome", "Color"]}] -> [_ _ _ _ _ w296]
          frame Default {
            w254 = FALSE ("Visible")
            w253 = FALSE ("Visible")
            n136 = property on="Motor" class="Clust (strict)"("Visible"=w253) -> ()  [unwired: 2 in, 2 out]
            n137 = property on="Test Ring" class="Ring (strict)"("Visible"=w253) -> ()  [unwired: 2 in, 2 out]
            n138 = property on="Rev/Fwd" class="Clust (strict)"("Visible"=w254) -> ()  [unwired: 2 in, 2 out]
            n139 = property on="On/Off" class="Bool (strict)"("Visible"=w254) -> ()  [unwired: 2 in, 2 out]
            n140 = property on="Test Slider" class="Slide (strict)"("Visible"=w254) -> ()  [unwired: 2 in, 2 out]
          }
          frame "Analog Out", "Motor", "PWM" {
            w260 = FALSE ("Visible")
            n141 = case shown="\"Analog Out\"" w259 {
              tunnel: [1.0 ("Value") -1.0 ("Value") 0.0 ("Value")] -> w258
              tunnel: [255.0 ("Value") 1.0 ("Value") 5.0 ("Value")] -> w257
              tunnel: [128.0 ("Value") 0.0 ("Value") 0.0 ("Value")] -> w256
              tunnel: [64.0 ("Value") 0.5 ("Value") 1.0 ("Value")] -> w255
              frame "PWM" {
              }
              frame "Motor", Default {
              }
              frame "Analog Out" {
              }
            }
            n142 = property on="Motor" class="Clust (strict)"("Visible"=TRUE) -> ()  [unwired: 2 in, 2 out]
            n143 = property on="Value" class="Slide (strict)"("Value"=w256, "Scale.Minimum"=w258, "Scale.Maximum"=w257, "Scale.Increment"=w255) -> ()  [unwired: 2 in, 2 out]
            n144 = property on="On/Off" class="Bool (strict)"("Visible"=w260) -> ()  [unwired: 2 in, 2 out]
            n145 = property on="Test Slider" class="Slide (strict)"("Visible"=w260) -> ()  [unwired: 2 in, 2 out]
            n146 = property on="Test Ring" class="Ring (strict)"("Visible"=w260) -> ()  [unwired: 2 in, 2 out]
            n147 = property on="Rev/Fwd" class="Clust (strict)"("Visible"=w260) -> ()  [unwired: 2 in, 2 out]
          }
          frame "Servo" {
            w276 = FALSE ("Visible")
            n148 = call <vilib>:"NT Read Number.vi"("Name"=w278) -> ("Numeric"=w277:dbl)  [unwired: 9 in, 1 out]
            n149 = property on="Test Slider" class="Slide (strict)"("Visible"=TRUE, "Scale.Maximum"=170.0 ("Scale.Range:Maximum")) -> ()  [unwired: 2 in, 2 out]
            n150 = local write "Test Slider"(w277) -> ()
            n151 = property on="Motor" class="Clust (strict)"("Visible"=w276) -> ()  [unwired: 2 in, 2 out]
            n152 = property on="Rev/Fwd" class="Clust (strict)"("Visible"=w276) -> ()  [unwired: 2 in, 2 out]
            n153 = property on="On/Off" class="Bool (strict)"("Visible"=w276) -> ()  [unwired: 2 in, 2 out]
            n154 = property on="Test Ring" class="Ring (strict)"("Visible"=w276) -> ()  [unwired: 2 in, 2 out]
          }
          frame "Relay", "Solenoid" {
            w279 = FALSE ("Visible")
            n155 = property on="Motor" class="Clust (strict)"("Visible"=w279) -> ()  [unwired: 2 in, 2 out]
            n156 = property on="Test Slider" class="Slide (strict)"("Visible"=w279) -> ()  [unwired: 2 in, 2 out]
            n157 = Search and Replace String(input string=w280, search string="/Value  **", replace string="/Direction") -> (result string=w286:string)  [unwired: 5 in, 3 out]
            n158 = property on="Test Ring" class="Ring (strict)"("Visible"=w279) -> ()  [unwired: 2 in, 2 out]
            n159 = call <vilib>:"NT Read String.vi"("Name"=w286) -> ("String"=w284:string)  [unwired: 9 in, 1 out]
            n160 = Equal?(x="Both directions", y=w284) -> (x = y?=w282:bool)
            n161 = Not(x=w282) -> (.not. x?=w283:bool)
            n162 = property on="Rev/Fwd" class="Clust (strict)"("Visible"=w282) -> ()  [unwired: 2 in, 2 out]
            n163 = property on="On/Off" class="Bool (strict)"("Visible"=w283, "Caption.Text"=w281) -> ()  [unwired: 2 in, 2 out]
          }
          frame "Compressor", "Digital Out" {
            w289 = FALSE ("Visible")
            # "Get direction and finish"
            n164 = property on="Motor" class="Clust (strict)"("Visible"=w289) -> ()  [unwired: 2 in, 2 out]
            n165 = property on="Test Slider" class="Slide (strict)"("Visible"=w289) -> ()  [unwired: 2 in, 2 out]
            n166 = property on="Test Ring" class="Ring (strict)"("Visible"=w289) -> ()  [unwired: 2 in, 2 out]
            n167 = property on="On/Off" class="Bool (strict)"("Visible"=TRUE, "Caption.Text"=w290) -> ()  [unwired: 2 in, 2 out]
            n168 = property on="Rev/Fwd" class="Clust (strict)"("Visible"=FALSE) -> ()  [unwired: 2 in, 2 out]
          }
          frame "Camera" {
            n169 = call <vilib>:"Get Last Path Segment.vi"("String in"=w297) -> ("String out"=w298:string)  [unwired: 10 in]
            n170 = property on="On/Off" class="Bool (strict)"("Visible"=FALSE) -> ()  [unwired: 2 in, 2 out]
            n171 = property on="Motor" class="Clust (strict)"("Visible"=FALSE) -> ()  [unwired: 2 in, 2 out]
            n172 = property on="Rev/Fwd" class="Clust (strict)"("Visible"=FALSE) -> ()  [unwired: 2 in, 2 out]
            n173 = case shown="\"White Balance  **\"" w298 {
              tunnel: w297 -> [w304 w313 w322 w331 w340 _ w346]
              tunnel: w296 -> [w302 w310 w319 w328 w337 _ _]
              frame "Size  **" {
                n174 = Index Array(array=w302) -> (element=w301:cluster{string[]})  [unwired: 1 in]
                n175 = call <vilib>:"NT Read String.vi"("Name"=w304) -> ("String"=w303:string)  [unwired: 9 in, 1 out]
                n176 = Unbundle(w301) -> (w299:string[])
                n177 = Match First String(2:w299, 3:w303) -> (0:w300:i32)  [unwired: 1 out]
                n178 = property on="Test Ring" class="Ring (strict)"("Value"=w300, "Strings []"=w299) -> ()  [unwired: 2 in, 2 out]
                n179 = property on="Test Ring" class="Ring (strict)"("Visible"=TRUE) -> ()  [unwired: 2 in, 2 out]
                n180 = property on="Test Slider" class="Slide (strict)"("Visible"=FALSE) -> ()  [unwired: 2 in, 2 out]
              }
              frame "White Balance  **" {
                n181 = Index Array(array=w310, index=1) -> (element=w311:cluster{string[]})
                n182 = call <vilib>:"NT Read String.vi"("Name"=w313) -> ("String"=w312:string)  [unwired: 9 in, 1 out]
                n183 = Unbundle(w311) -> (w308:string[])
                n184 = Match First String(2:w308, 3:w312) -> (0:w307:i32)  [unwired: 1 out]
                n185 = property on="Test Ring" class="Ring (strict)"("Value"=w307, "Strings []"=w308) -> ()  [unwired: 2 in, 2 out]
                n186 = property on="Test Ring" class="Ring (strict)"("Visible"=TRUE) -> ()  [unwired: 2 in, 2 out]
                n187 = property on="Test Slider" class="Slide (strict)"("Visible"=FALSE) -> ()  [unwired: 2 in, 2 out]
              }
              frame "Exposure  **" {
                n188 = Index Array(array=w319, index=2) -> (element=w320:cluster{string[]})
                n189 = call <vilib>:"NT Read String.vi"("Name"=w322) -> ("String"=w321:string)  [unwired: 9 in, 1 out]
                n190 = Unbundle(w320) -> (w316:string[])
                n191 = Match First String(2:w316, 3:w321) -> (0:w317:i32)  [unwired: 1 out]
                n192 = property on="Test Ring" class="Ring (strict)"("Value"=w317, "Strings []"=w316) -> ()  [unwired: 2 in, 2 out]
                n193 = property on="Test Ring" class="Ring (strict)"("Visible"=TRUE) -> ()  [unwired: 2 in, 2 out]
                n194 = property on="Test Slider" class="Slide (strict)"("Visible"=FALSE) -> ()  [unwired: 2 in, 2 out]
              }
              frame "Exposure Priority  **" {
                n195 = Index Array(array=w328, index=3) -> (element=w329:cluster{string[]})
                n196 = call <vilib>:"NT Read String.vi"("Name"=w331) -> ("String"=w330:string)  [unwired: 9 in, 1 out]
                n197 = Unbundle(w329) -> (w325:string[])
                n198 = Match First String(2:w325, 3:w330) -> (0:w326:i32)  [unwired: 1 out]
                n199 = property on="Test Ring" class="Ring (strict)"("Value"=w326, "Strings []"=w325) -> ()  [unwired: 2 in, 2 out]
                n200 = property on="Test Ring" class="Ring (strict)"("Visible"=TRUE) -> ()  [unwired: 2 in, 2 out]
                n201 = property on="Test Slider" class="Slide (strict)"("Visible"=FALSE) -> ()  [unwired: 2 in, 2 out]
              }
              frame "Color Enable  **" {
                n202 = Index Array(array=w337, index=4) -> (element=w338:cluster{string[]})
                n203 = call <vilib>:"NT Read String.vi"("Name"=w340) -> ("String"=w339:string)  [unwired: 9 in, 1 out]
                n204 = Unbundle(w338) -> (w334:string[])
                n205 = Match First String(2:w334, 3:w339) -> (0:w335:i32)  [unwired: 1 out]
                n206 = property on="Test Ring" class="Ring (strict)"("Value"=w335, "Strings []"=w334) -> ()  [unwired: 2 in, 2 out]
                n207 = property on="Test Ring" class="Ring (strict)"("Visible"=TRUE) -> ()  [unwired: 2 in, 2 out]
                n208 = property on="Test Slider" class="Slide (strict)"("Visible"=FALSE) -> ()  [unwired: 2 in, 2 out]
              }
              frame Default {
                n209 = property on="Test Ring" class="Ring (strict)"("Visible"=FALSE) -> ()  [unwired: 2 in, 2 out]
                n210 = property on="Test Slider" class="Slide (strict)"("Visible"=FALSE) -> ()  [unwired: 2 in, 2 out]
              }
              frame "Brightness  **", "Color Level  **", "Compression  **", "FPS  **", "Sharpness  **" {
                n211 = call <vilib>:"NT Read Number.vi"("Name"=w346) -> ("Numeric"=w345:dbl)  [unwired: 9 in, 1 out]
                n212 = local write "Test Slider"(w345) -> ()
                n213 = property on="Test Slider" class="Slide (strict)"("Visible"=TRUE, "Scale.Maximum"=100.0 ("Scale.Range:Maximum")) -> ()  [unwired: 2 in, 2 out]
                n214 = property on="Test Ring" class="Ring (strict)"("Visible"=FALSE) -> ()  [unwired: 2 in, 2 out]
              }
            }
          }
        }
        n215 = property on="Progress" class="Clust (strict)"("Visible"=FALSE) -> ()  [unwired: 2 in, 2 out]
      }
      event "Test Name": Mouse Enter {
        # "Populate the ring with the list of tests"
        n216 = event-data() -> ()  [unwired: 1 in, 1 out]
        n217 = call <vilib>:"NT Read String Array.vi"("Name"="TestMode/TestList") -> ("String Array"=w354:string[])  [unwired: 9 in, 1 out]
        n218 = Build Array (concatenate)("Select the test to run...", w354) -> (w353:string[])
        n219 = property on="Test Name" class="Ring (strict)"("Strings []"=w353) -> ()  [unwired: 2 in, 2 out]
      }
      event "Test Name": Value Change {
        w356 = FALSE ("Visible")
        # "Tell the robot the test name to run"
        n220 = event-data() -> ("NewVal"=w360:u16)  [unwired: 1 in]
        n221 = property on="Test Name" class="Ring (strict)"() -> ("Strings []"=w361:string[])  [unwired: 2 in, 2 out]
        n222 = local write "Progress"(T6 {"Test Progress"=0, "Test Progress Text"=""} ("Progress")) -> ()
        n223 = Index Array(array=w361, index=w360) -> (element=w359:string)
        n224 = call <vilib>:"NT Write String.vi"("String"=w359, "Name"="TestMode/TestName") -> ()  [unwired: 9 in, 1 out]
        n225 = property on="Progress" class="Clust (strict)"("Visible"=TRUE) -> ()  [unwired: 2 in, 2 out]
        n226 = property on="Motor" class="Clust (strict)"("Visible"=w356) -> ()  [unwired: 2 in, 2 out]
        n227 = property on="Test Slider" class="Slide (strict)"("Visible"=w356) -> ()  [unwired: 2 in, 2 out]
        n228 = property on="On/Off" class="Bool (strict)"("Visible"=w356) -> ()  [unwired: 2 in, 2 out]
        n229 = property on="Rev/Fwd" class="Clust (strict)"("Visible"=w356) -> ()  [unwired: 2 in, 2 out]
        n230 = property on="Test Ring" class="Ring (strict)"("Visible"=w356) -> ()  [unwired: 2 in, 2 out]
      }
      event "Select Auto": Mouse Enter {
        # "Populate the combo box with the list of autonomous options"
        n231 = event-data() -> ()  [unwired: 1 in, 1 out]
        n232 = call <vilib>:"NT Read String Array.vi"("Name"="Auto List") -> ("String Array"=w363:string[])  [unwired: 9 in, 1 out]
        n233 = property on="Select Auto" class="CmbBox"("Strings[]"=w363) -> ()  [unwired: 2 in, 2 out]
      }
      event "Select Auto": Value Change {
        # "User modified the Auto Selection. Write to NT variable so robot knows."
        n234 = event-data() -> ("NewVal"=w366:string)  [unwired: 1 in]
        n235 = call <vilib>:"NT Write String.vi"("String"=w366, "Name"="Auto Selector") -> ()  [unwired: 9 in, 1 out]
      }
      event "Command Selection": Value Change {
        # "Get the params and show in table"
        n236 = event-data() -> ("NewVal"=w372:i32)  [unwired: 1 in]
        n237 = property on="Command Selection" class="MCListbox (strict)"() -> ("ItemNames"=w370:string[][])  [unwired: 2 in, 2 out]
        n238 = call <vilib>:"WPI_DashboardUpdate Command Params.vi"("NewVal"=w372, "Commands"=w370, "Param Tbl"=w371) -> ()  [unwired: 8 in, 1 out]
      }
      event "Execute Command": Value Change {
        # "Started one, Unique ID holds\nresponse"
        n239 = event-data() -> ()  [unwired: 1 in, 1 out]
        n240 = property on="Command Selection" class="MCListbox (strict)"() -> ("ItemNames"=w383:string[][])  [unwired: 2 in, 2 out]
        n241 = Index Array(array=w383, index (row)="Command Selection", index (col)=0) -> (element=w381:string)
        n242 = call <vilib>:"Invoke Commands.vi"("Command Params"="Command Params", "Function Name"=w381) -> ("Params"=w377:u8, "Started"=w376:bool)  [unwired: 7 in, 1 out]
        n243 = Array Subset(array="Command Params", length (row)=w377) -> (w378:string[][])  [unwired: 3 in]
        n244 = Select(t="Executing" ("Cmd Status"), s=w376, f="" ("Cmd Status")) -> (s? t:f=→"Cmd Status":string)
      }
      event "Command Selection": Double Click {
        n245 = event-data() -> ("Row"=w391:i32)  [unwired: 1 in]
        n246 = property on="Command Selection" class="MCListbox (strict)"() -> ("ItemNames"=w394:string[][])  [unwired: 2 in, 2 out]
        n247 = local read "Command Params"() -> (w390:string[][])
        n248 = Index Array(array=w394, index (row)=w391, index (col)=0) -> (element=w392:string)
        n249 = call <vilib>:"Invoke Commands.vi"("Command Params"=w390, "Function Name"=w392) -> ("Params"=w389:u8, "Started"=w384:bool)  [unwired: 7 in, 1 out]
        n250 = Array Subset(array=w390, length (row)=w389) -> (w388:string[][])  [unwired: 3 in]
        n251 = Select(t="Executing" ("Cmd Status"), s=w384, f="" ("Cmd Status")) -> (s? t:f=w385:string)
        n252 = local write "Cmd Status"(w385) -> ()
      }
      event "CheckList": Double Click {
        # "Shift clears all"
        # "Update symbols on the listbox"
        n253 = event-data() -> ("PlatMods.Shift"=w396:bool, "Row"=w398:i32)  [unwired: 1 in]
        n254 = case shown="True" w396 {
          tunnel: w398 -> [w402 _]
          tunnel: 1 -> [w401 _]
          frame False {
            n255 = property on="CheckList" class="LstBox (strict)"() -> ("Item Symbols"=w400:i32[])  [unwired: 2 in, 2 out]
            n256 = Replace Array Subset(array=w400, new element=w401, index=w402) -> (w399:i32[])
            n257 = property on="CheckList" class="LstBox (strict)"("Item Symbols"=w399) -> ()  [unwired: 2 in, 2 out]
          }
          frame True {
            w403 = 0 ("Top Row")
            n258 = property on="CheckList" class="LstBox (strict)"() -> ("Number of Rows"=w405:u32)  [unwired: 2 in, 2 out]
            n259 = Initialize Array(0, w405) -> (w404:i32[])
            n260 = property on="CheckList" class="LstBox (strict)"("Top Row"=w403, "Value"=w403, "Item Symbols"=w404) -> ()  [unwired: 2 in, 2 out]
          }
        }
      }
      event "CheckList": Key Down {
        # "Update symbols on the listbox\nLeft and right keys check and uncheck"
        n261 = event-data() -> ("VKey"=w409:T23)  [unwired: 1 in]
        n262 = case shown="\"Left\", \"Right\"" w409 {
          selector: w409 -> [w414 _]
          tunnel: eventvkey."Left" ("VKey") -> [w412 _]
          frame "Left", "Right" {
            n263 = Equal?(x=w412, y=w414) -> (x = y?=w413:bool)
            n264 = Select(t=0, s=w413, f=1) -> (s? t:f=w415:i32)
            n265 = property on="CheckList" class="LstBox (strict)"() -> ("Item Symbols"=w418:i32[])  [unwired: 2 in, 2 out]
            n266 = Replace Array Subset(array=w418, new element=w415, index="CheckList") -> (w417:i32[])
            n267 = property on="CheckList" class="LstBox (strict)"("Item Symbols"=w417) -> ()  [unwired: 2 in, 2 out]
          }
          frame Default {
          }
        }
      }
      event "Motor.Enable": Value Change {
        # "When the test mode otor enable helper is set, update that\ntree row item's value"
        n268 = event-data() -> ("NewVal"=w424:bool)  [unwired: 1 in]
        n269 = Unbundle("Motor") -> ("Value"=w423:dbl)  [unwired: 1 out]
        n270 = Select(t=w423, s=w424, f=0.0) -> (s? t:f=w421:dbl)
        n271 = call <vilib>:"NT Write Number.vi"("Numeric"=w421, "Name"=w420) -> ()  [unwired: 9 in, 1 out]
      }
      event "Test Slider": Value Change {
        # "When the test mode slider helper is set, update that\ntree row item's value"
        n272 = event-data() -> ("NewVal"=w427:dbl)  [unwired: 1 in]
        n273 = call <vilib>:"NT Write Number.vi"("Numeric"=w427, "Name"=w428) -> ()  [unwired: 9 in, 1 out]
      }
      event "On/Off": Value Change {
        # "When the test mode on/off helper value is set, update that\ntree row item's value"
        n274 = event-data() -> ("NewVal"=w432:bool)  [unwired: 1 in]
        n275 = Boolean To (0,1)(Boolean=w432) -> (0, 1=w431:i16)
        n276 = call <vilib>:"NT Write Number.vi"("Numeric"=w431, "Name"=w430) -> ()  [unwired: 9 in, 1 out]
      }
      event "Rev/Fwd": Value Change {
        # "When the test mode helper value for relays is set, update that\ntree row item's value"
        n277 = event-data() -> ("NewVal.Forward"=w440:bool, "NewVal.Reverse"=w439:bool)  [unwired: 1 in]
        n278 = Boolean To (0,1)(Boolean=w440) -> (0, 1=w436:i16)
        n279 = Boolean To (0,1)(Boolean=w439) -> (0, 1=w438:i16)
        n280 = Negate(x=w438) -> (-x=w437:i16)
        n281 = Add(x=w436, y=w437) -> (x+y=w435:i16)
        n282 = call <vilib>:"NT Write Number.vi"("Numeric"=w435, "Name"=w434) -> ()  [unwired: 9 in, 1 out]
      }
      event "Test Ring": Value Change {
        # "When a test mode helper value is selected from the ring,\nset the tree item's variable to the string value"
        n283 = event-data() -> ("NewVal"=w444:u16)  [unwired: 1 in]
        n284 = property on="Test Ring" class="Ring (strict)"() -> ("Strings []"=w445:string[])  [unwired: 2 in, 2 out]
        n285 = Index Array(array=w445, index=w444) -> (element=w443:string)
        n286 = call <vilib>:"NT Write String.vi"("String"=w443, "Name"=w442) -> ()  [unwired: 9 in, 1 out]
      }
      event "Rec Mode": Value Change {
        # "Update globals for recording mode and path to read log from.\nClear when logging and let NetworkTables set path for vision to\nuse."
        n287 = event-data() -> ("NewVal"=w456:enum32{"Stop", "Record", "Playback"})  [unwired: 1 in]
        n288 = global write "WPI_DashboardLogging Global.vi" "Logging Filename"(path "") -> ()
        n289 = global write "WPI_DashboardLogging Global.vi" "Recording"(w456) -> ()
        n290 = case shown="\"Playback\"" w456 {
          tunnel: w455 -> [_ w458 w467]
          tunnel: [_ _ w466] -> w453
          tunnel: [_ _ w465] -> _
          tunnel: w451 -> [_ _ w463]
          tunnel: cluster{i32, i32} {-250, 170} -> [_ _ w462]
          tunnel: [_ _ T24 {"Image Size"=TRUE, "Image Type"=TRUE, "Pixel Value"=TRUE, "ROI Information"=TRUE, "Zoom Factor"=FALSE} ("Image Information Shown:All Elements")] -> w446
          tunnel: [_ _ TRUE ("Zoom Factor")] -> w447
          tunnel: w449 -> [_ _ w459]
          frame Default {
          }
          frame "Stop", "Record" {
            # "Place Window too"
            n291 = invoke class="VI" method="FP.Close"(reference=w458) -> (reference out=w457:refnum<vi>)  [unwired: 2 in, 2 out]
            n292 = invoke class="VI" method="Abort VI"(reference=w457) -> ()  [unwired: 2 in, 3 out]
          }
          frame "Playback" {
            n293 = call "Open Playback Panel.vi"("Offset"=w462, "DB VI Ref"=w463, "Playback in"=w467) -> ("Playback out"=w464:refnum<vi>)  [unwired: 8 in]
            n294 = register-events(w464, w459) -> (reference out=w466:refnum<event-registration>, error out=w465:errorcluster)  [unwired: 2 in]
          }
        }
        n295 = property on="Camera Image Right" class="ImageControl"("Image Information Shown"=w446, "Image Information Visible"=w447) -> ()  [unwired: 2 in, 2 out]
        n296 = property on="Camera Image" class="ImageControl"("Image Information Shown"=w446, "Image Information Visible"=w447) -> ()  [unwired: 2 in, 2 out]
        n297 = call <vilib>:"WPI_DashboardNT Log FieldName Cache.vi"("Operation"=enum16{"Lookup/Add", "Index", "Clear"}."Clear") -> ()  [unwired: 8 in, 3 out]
      }
      event Panel Close {
        w469 = enum32{"Stop", "Record", "Playback"}."Stop" ("Rec Mode")
        # "Playback window has been closed, abort"
        n298 = event-data() -> ()  [unwired: 1 in, 4 out]
        n299 = local write "Rec Mode"(w469) -> ()
        n300 = global write "WPI_DashboardLogging Global.vi" "Recording"(w469) -> ()
      }
      event Panel Close {
        # "Abort playback window and ourself"
        n301 = event-data() -> ()  [unwired: 1 in, 4 out]
        n302 = invoke class="VI" method="FP.Close"(reference=w473) -> (reference out=w472:refnum<vi>)  [unwired: 2 in, 2 out]
        n303 = invoke class="VI" method="Abort VI"(reference=w472) -> (error out=w471:errorcluster)  [unwired: 2 in, 2 out]
        n304 = invoke class="VI" method="Abort VI"(error in=w471) -> ()  [unwired: 2 in, 3 out]
      }
      event User Event {
        n305 = event-data() -> ("IDs"=w480:cluster{"RPC field ID":u16, "Unique ID":u16}, "String"=w479:string)  [unwired: 1 in]
        n306 = Bundle("IDs"=w480, "String"=w479) -> (w478:T10)  [unwired: 1 in]
        n307 = call <vilib>:"Retrieve RPC Response.vi"("RPC Response"=w478) -> ("Output"=w476:string[][])  [unwired: 10 in]
        n308 = Build Array (concatenate)(w474, w476) -> (w475:string[][])
        n309 = local write "Command Params"(w475) -> ()
        n310 = local write "Cmd Status"("" ("Cmd Status")) -> ()
      }
      event "Tree": Double Click {
        n311 = event-data() -> ("PlatMods"=w486:T27, "Tag"=w483:string)  [unwired: 1 in]
        n312 = Unbundle(w486) -> ("Shift"=w485:bool)  [unwired: 4 out]
        n313 = String Subset(string=w483, length (rest)=1 ("length (rest)")) -> (substring=w482:string)  [unwired: 1 in]
        n314 = Not(x=w485) -> (.not. x?=w484:bool)
        n315 = case shown="\"/\"" w482 {
          tunnel: w483 -> [_ w489]
          tunnel: w484 -> [_ w488]
          frame Default {
          }
          frame "/" {
            n316 = call <vilib>:"NT Update Persistence.vi"("Persistence"=w488, "Name"=w489) -> ()  [unwired: 9 in, 1 out]
          }
        }
      }
    }
  }
  n317 = while {
    tunnel: w65 -> [w491]
    i -> [w494]
    stop <- FALSE stop-if-true
    n318 = Wait (ms)(milliseconds to wait=u32 100) -> ()  [unwired: 1 out]
    n319 = case shown="\"Playback\"" "Rec Mode" {
      tunnel: w494 -> [_ _ w509]
      tunnel: [u32 2829099 ("Base Color") u32 11141120 ("Target Color") w498] -> w490
      frame "Stop", Default {
        # "Reset the color, extra updates don't cost much"
      }
      frame "Record" {
      }
      frame "Playback" {
        # "Playback"
        n320 = Quotient & Remainder(x=w509, y=u32 50 ("milliseconds to wait")) -> (x-y*floor(x/y)=w505:u32)  [unwired: 1 out]
        n321 = Divide(x=w505, y=u32 50 ("milliseconds to wait")) -> (x/y=w502:dbl)
        n322 = Multiply(x=6.283185307179586, y=w502) -> (x*y=w507:dbl)
        n323 = Sine(x=w507) -> (sin(x)=w506:dbl)
        n324 = Absolute Value(x=w506) -> (abs(x)=w499:dbl)
        n325 = call "Interpolate RGB Color.vi"("Proportion"=w499, "Target Color"=u32 30976, "Base Color"=u32 2829099) -> ("Result Color"=w498:u32)  [unwired: 8 in]
      }
    }
    n326 = property class="Pane"(reference=w491, "PaneColor"=w490) -> ()  [unwired: 1 in, 2 out]
  }
  n327 = local write "Dashboard Tab"(T2."Operation" ("Dashboard Tab")) -> ()
  n328 = property on="On/Off" class="Bool (strict)"("Visible"=w36) -> ()  [unwired: 2 in, 2 out]
  n329 = property on="Motor" class="Clust (strict)"("Visible"=w36) -> ()  [unwired: 2 in, 2 out]
  n330 = property on="Progress" class="Clust (strict)"("Visible"=w36) -> ()  [unwired: 2 in, 2 out]
  n331 = property on="Test Ring" class="Ring (strict)"("Visible"=w36) -> ()  [unwired: 2 in, 2 out]
  n332 = property on="Rev/Fwd" class="Clust (strict)"("Visible"=w36) -> ()  [unwired: 2 in, 2 out]
  n333 = while {
    tunnel: u16 1741 ("timeout ms (25000)") -> [w511]
    stop <- FALSE stop-if-true
    n334 = TCP Create Listener(10:w511) -> (0:w510:errorcluster, 3:w512:refnum<k5>)  [unwired: 4 in, 1 out]
    n335 = case shown="No Error" w510 {
      selector: w510 -> [w514 _]
      tunnel: w512 -> [w515 _]
      frame No Error {
        n336 = while {
          tunnel: w515 -> [w518]
          tunnel: w514 -> [w517]
          stop <- FALSE stop-if-true
          n337 = TCP Wait On Listener(8:w517, 11:w518) -> (0:w519:errorcluster, 4:w520:refnum<k5>)  [unwired: 2 in, 3 out]
          n338 = local write "TCP"(w520) -> ()
          n339 = case shown="No Error" w519 {
            frame No Error {
            }
            frame Error {
              n340 = Wait (ms)(milliseconds to wait=u32 1000) -> ()  [unwired: 1 out]
            }
          }
        }
      }
      frame Error {
        n341 = Wait (ms)(milliseconds to wait=u32 1000) -> ()  [unwired: 1 out]
      }
    }
  }
  n342 = local write "Command Selection"(u16 0 ("milliseconds to wait")) -> ()
  n343 = local write "Command Params"(string[][] [] ("Command Params")) -> ()
  n344 = global write "WPI_DashboardLogging Global.vi" "Recording"(w59) -> ()
  n345 = local write "Rec Mode"(w59) -> ()
  n346 = call <vilib>:"NT Write String.vi"("String"="Select Auto", "Name"="Auto Selector") -> ()  [unwired: 9 in, 1 out]
  n347 = while {
    stop <- FALSE stop-if-true
    # "I/O Tab"
    n348 = call-poly <vilib>:"NT Read Value.vi"("Default Value"=0.0, "Name"="Top RPM") -> ("Numeric"=w529:dbl)  [unwired: 8 in, 1 out]
    n349 = Round To Nearest(number=w529) -> (nearest integer value=→"Top RPM":dbl)
    n350 = call-poly <vilib>:"NT Read Value.vi"("Default Value"=0.0, "Name"="Bottom RPM") -> ("Numeric"=w525:dbl)  [unwired: 8 in, 1 out]
    n351 = Round To Nearest(number=w525) -> (nearest integer value=→"Bottom RPM":dbl)
    n352 = Wait (ms)(milliseconds to wait=u32 50) -> ()  [unwired: 1 out]
  }
  n353 = while {
    stop <- FALSE stop-if-true
    # "Limelight Tab"
    n354 = call-poly <vilib>:"NT Read Value.vi"("Name"="/limelight/ty") -> ("Numeric"=→"Offset Y":dbl)  [unwired: 9 in, 1 out]
    n355 = call-poly <vilib>:"NT Read Value.vi"("Name"="/limelight/tx") -> ("Numeric"=→"Offset X":dbl)  [unwired: 9 in, 1 out]
    n356 = call-poly <vilib>:"NT Read Value.vi"("Name"="/limelight/ts") -> ("Numeric"=→"Skew":dbl)  [unwired: 9 in, 1 out]
    n357 = call-poly <vilib>:"NT Read Value.vi"("Name"="/limelight/ta") -> ("Numeric"=→"Area":dbl)  [unwired: 9 in, 1 out]
    n358 = Wait (ms)(milliseconds to wait=u32 50) -> ()  [unwired: 1 out]
  }
